vi "ble_rsp_gap_connect_direct.vi"(8 "error in (no error)":errorcluster, 11 "COM Bluegiga in":refnum<visa-resource-name>) -> (0 "error out":errorcluster, 2 "full message package":u8[](array[numeric]), 3 "COM Bluegiga out":refnum<visa-resource-name>)   [LabVIEW 2015]
uses:
  type_def/message_class.ctl
panel:
  out "success?":bool
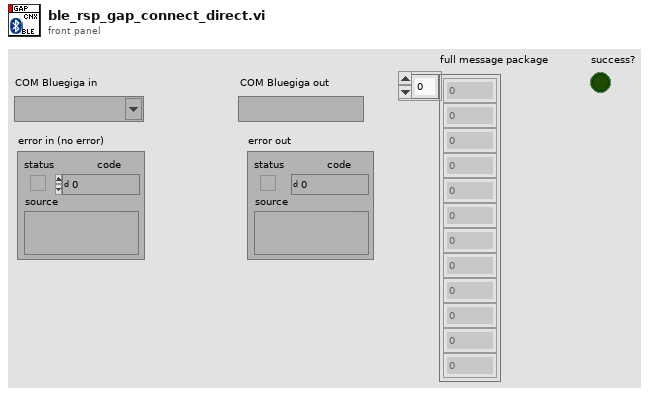
[diagram p1: front panel]
types:
  T1 = typedef "message_class.ctl" = u8
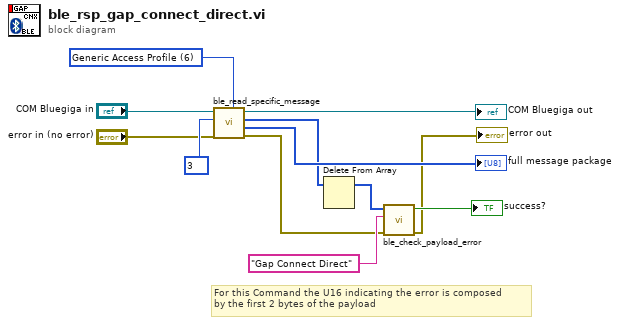
[diagram p0: block diagram]
diagram:
  w12 = T1 6 items=["System", "Persistent Store", "Attribute database", "Connection", "Attribute client", "Security Manager", "Generic Access Profile", "Hardware"] ("Command Class (System)")
  # "For this Command the U16 indicating the error is composed\nby the first 2 bytes of the payload"
  n1 = call "ble_read_specific_message.vi"("Command Class (System)"=w12, "error in (no error)"="error in (no error)", "Message ID (0x00)"=u8 3, "COM Bluegiga in"="COM Bluegiga in") -> ("error out"=w5:errorcluster, "full message package"=→"full message package":u8[], "specific payload"=w4:u8[], "COM Bluegiga out"=→"COM Bluegiga out":refnum<visa-resource-name>)  [unwired: 3 in, 1 out]
  n2 = Delete From Array(array=w4) -> (array with subset deleted=w3:u8[])  [unwired: 2 in, 1 out]
  n3 = call "ble_check_payload_error.vi"("error in (no error)"=w5, "error source"="Gap Connect Direct", "payload"=w3) -> ("error out"=→"error out":errorcluster, "success?"=→"success?":bool)  [unwired: 7 in]
